vi "MEMR-Initialize Reanalysis.vi"(0 "Path":path=path "D:/Data/MEMR/Ken/SFMH41-MEMR-1.txt", 5 "Params":T1, 11 "error in":errorcluster) -> (4 "Path dup":path=path "D:/Data/MEMR/Ken/SFMH41-MEMR-1.txt", 6 "Params (dup)":T1, 8 "State":T8, 15 "error out":errorcluster)   [LabVIEW 2020]
uses:
  Typedefs/MEMR-Params.ctl
  Typedefs/MEMR-Probe.ctl
  Typedefs/MEMR-Elicitor.ctl
  Human Studies/SFM Frontend/LV Source/Typedefs/HSTS-Transducer.ctl
  Typedefs/MEMR-Sequence.ctl
  Typedefs/MEMR-Analysis.ctl
  Typedefs/MEMR-Timing.ctl
  Typedefs/MEMR-Analysis State.ctl
  Utility VIs/Math VIs/dB to Linear (scalar).vi
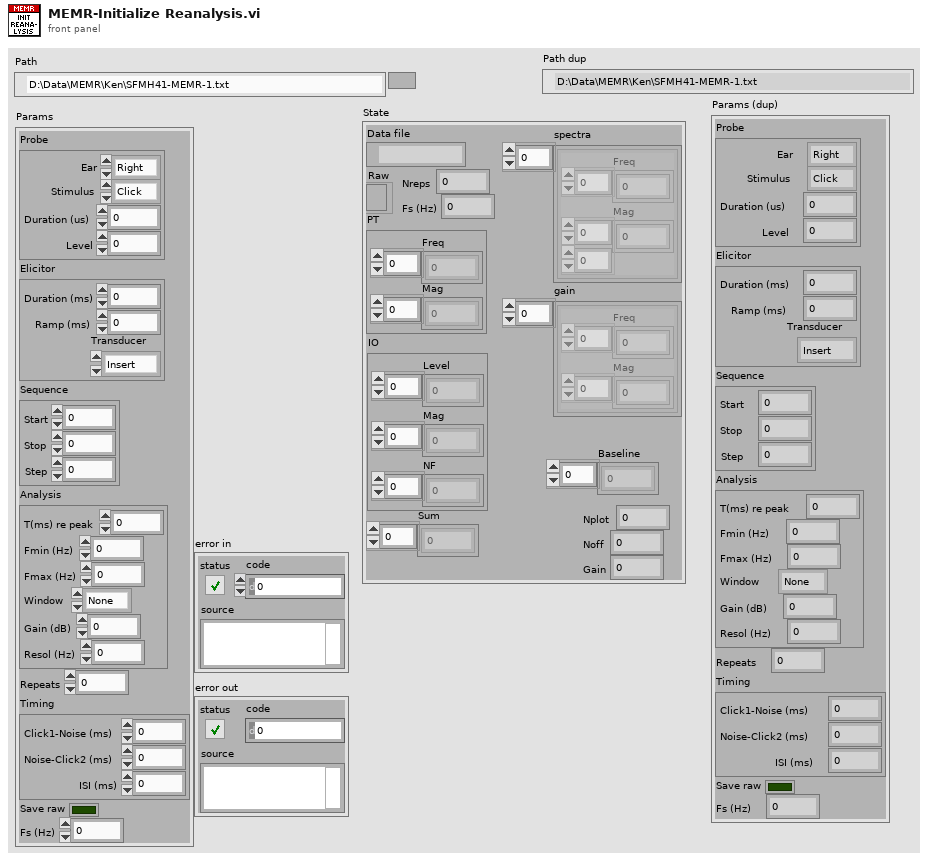
[diagram p1: front panel]
types:
  T1 = typedef "MEMR-Params.ctl" = cluster{"Probe":T2, "Elicitor":T3, "Sequence":T5, "Analysis":T6, "Repeats":i32, "Timing":T7, "Save raw":bool, "Fs (Hz)":dbl}
  T2 = typedef "MEMR-Probe.ctl" = cluster{"Ear":enum16{"Right", "Left"}, "Stimulus":enum16{"Click", "Chirp"}, "Duration (us)":dbl, "Level":dbl}
  T3 = typedef "MEMR-Elicitor.ctl" = cluster{"Duration (ms)":dbl, "Ramp (ms)":dbl, "Transducer":T4}
  T4 = typedef "HSTS-Transducer.ctl" = enum16{"Insert", "TDH-39", "HD300", "ER-10X"}
  T5 = typedef "MEMR-Sequence.ctl" = cluster{"Start":dbl, "Stop":dbl, "Step":dbl}
  T6 = typedef "MEMR-Analysis.ctl" = cluster{"T(ms) re peak":dbl, "Fmin (Hz)":dbl, "Fmax (Hz)":dbl, "Window":enum16{"None", "Hanning", "Hamming"}, "Gain (dB)":dbl, "Resol (Hz)":dbl}
  T7 = typedef "MEMR-Timing.ctl" = cluster{"Click1-Noise (ms)":dbl, "Noise-Click2 (ms)":dbl, "ISI (ms)":dbl}
  T8 = typedef "MEMR-Analysis State.ctl" = cluster{"Data file":path, "Raw":refnum<file>, "PT":cluster{"Freq":dbl[], "Mag":dbl[]}, "IO":cluster{"Level":dbl[], "Mag":dbl[], "NF":dbl[]}, "Nreps":i32, "Fs (Hz)":dbl, "Sum":dbl[], "Nplot":i32, "Noff":i32, "Gain":dbl, "spectra":cluster{"Freq":dbl[], "Mag":dbl[][]}[], "gain":cluster{"Freq":dbl[], "Mag":dbl[]}[], "Baseline":dbl[]}
  T9 = enum16{"open", "replace", "create", "open or create", "replace or create", "replace or create with confirmation"}
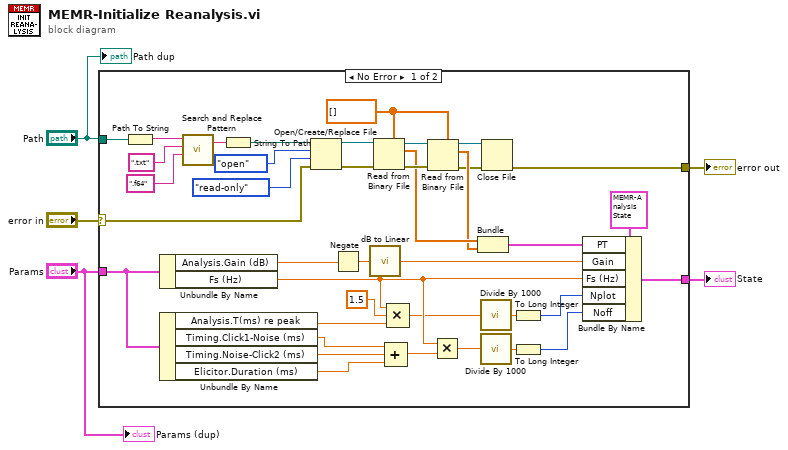
[diagram p0: block diagram]
diagram:
  n1 = case shown="No Error" "error in" {
    selector: "error in" -> [w6 w45]
    tunnel: "Path" -> [w12 _]
    tunnel: "Params" -> [w11 _]
    tunnel: [w10 _] -> w3
    tunnel: [w7 w45] -> w2
    frame No Error {
      w13 = dbl[] []
      n2 = Path To String(path=w12) -> (string=w44:string)
      n3 = Unbundle By Name(w11) -> ("Analysis.Gain (dB)"=w31:dbl, "Fs (Hz)"=w27:dbl)
      n4 = Unbundle By Name(w11) -> ("Analysis.T(ms) re peak"=w18:dbl, "Timing.Click1-Noise (ms)"=w22:dbl, "Timing.Noise-Click2 (ms)"=w23:dbl, "Elicitor.Duration (ms)"=w24:dbl)
      n5 = call <vilib>:"Search and Replace Pattern.vi"("string"=w44, "regular expression (\"\")"=".txt" ("regular expression (\"\")"), "replace string (\"\")"=".f64" ("replace string (\"\")")) -> ("result string"=w41:string)  [unwired: 2 in, 1 out]
      n6 = String To Path(string=w41) -> (path=w40:path)
      n7 = Open/Create/Replace File(file path (use dialog)=w40, error in=w6, operation (0:open)=T9."open", access (0:read/write)=enum16{"read/write", "read-only", "write-only"}."read-only") -> (refnum out=w36:refnum<file>, error out=w37:errorcluster)  [unwired: 2 in, 1 out]
      n8 = Negate(x=w31) -> (-x=w32:dbl)
      n9 = call-poly "dB to Linear.vi"("dB"=w32) -> ("linear"=w33:dbl)
      n10 = Read from Binary File(5:w13, 8:w37, 11:w36) -> (0:w35:errorcluster, 2:w15:dbl[], 3:w34:refnum<file>)  [unwired: 3 in, 1 out]
      n11 = Compound Arithmetic op=ADD(w22, w23, w24) -> (w25:dbl)
      n12 = Compound Arithmetic op=MULTIPLY(w27, 1.5 ("x"), w18) -> (w20:dbl)
      n13 = Read from Binary File(5:w13, 8:w35, 11:w34) -> (0:w8:errorcluster, 2:w14:dbl[], 3:w9:refnum<file>)  [unwired: 3 in, 1 out]
      n14 = Multiply(x=w27, y=w25) -> (x*y=w28:dbl)
      n15 = Bundle(w15, w14) -> (w16:cluster{dbl[], dbl[]})  [unwired: 1 in]
      n16 = call "Divide By 1000.vi"("X"=w20) -> ("X/1000"=w26:dbl)
      n17 = call "Divide By 1000.vi"("X"=w28) -> ("X/1000"=w29:dbl)
      n18 = Close File(refnum=w9, error in=w8) -> (error out=w7:errorcluster)  [unwired: 1 out]
      n19 = To Long Integer(number=w26) -> (32bit integer=w21:i32)
      n20 = To Long Integer(number=w29) -> (32bit integer=w30:i32)
      n21 = Bundle By Name(cluster=T8 {"Data file"=path "", "Raw"=refnum, "PT"={"Freq"=[], "Mag"=[]}, "IO"={"Level"=[], "Mag"=[], "NF"=[]}, "Nreps"=0, "Fs (Hz)"=0.0, "Sum"=[], "Nplot"=0, "Noff"=0, "Gain"=0.0, "spectra"=[], "gain"=[], "Baseline"=[]} ("Analysis State"), "PT"=w16, "Gain"=w33, "Fs (Hz)"=w27, "Nplot"=w21, "Noff"=w30) -> (w10:T8)
    }
    frame Error {
    }
  }
  "State" <- w3
  "error out" <- w2
  "Params (dup)" <- "Params"
  "Path dup" <- "Path"
